vi "Parse Unregister Message.vi"(0 "state":string, 1 "Module Name":string, 5 "args":string) -> (4 "target":string, 6 "source":string, 8 "status":string, 10 "api":string)   [LabVIEW 2017, in "Communicable State Machine.lvlib"]
uses:
  Communicable State Machine.lvlib
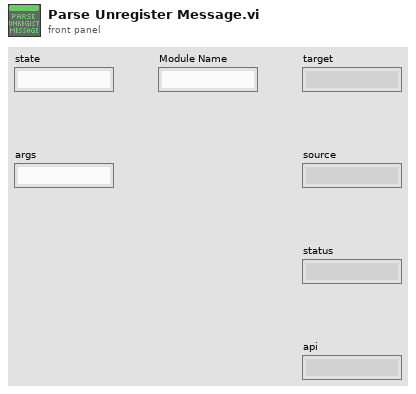
[diagram p1: front panel]
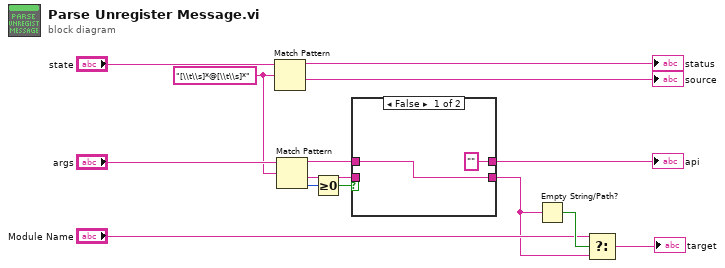
[diagram p0: block diagram]
diagram:
  w12 = "[\\t\\s]*@[\\t\\s]*" ("regular expression")
  n1 = Match Pattern(string="state", regular expression=w12) -> (before substring=→"status":string, after substring=→"source":string)  [unwired: 1 in, 2 out]
  n2 = Match Pattern(string="args", regular expression=w12) -> (before substring=w5:string, after substring=w9:string, offset past match=w7:i32)  [unwired: 1 in, 1 out]
  n3 = Greater Or Equal To 0?(x=w7) -> (x >= 0?=w8:bool)
  n4 = case shown="False" w8 {
    tunnel: w9 -> [_ w18]
    tunnel: [w15 w18] -> w1
    tunnel: ["" ("args") w17] -> w6
    tunnel: w5 -> [w15 w17]
    frame False {
    }
    frame True {
    }
  }
  "api" <- w6
  n5 = Empty String/Path?(string/path=w1) -> (empty?=w4:bool)
  n6 = Select(t="Module Name", s=w4, f=w1) -> (s? t:f=→"target":string)
